vi "Initialise Tree.vi"(8 "error in (no error)":errorcluster, 11 "Resource Directory":path) -> (0 "error out":errorcluster, 3 "Teapot":T1)   [LabVIEW 2022 SP3, in "Application.lvlib" / "Scene.lvclass"]
uses:
  Scene.lvclass
  Libraries/3D/Object.ctl
  Libraries/3D/Triangle 3D.ctl
  Libraries/3D/Vector 3D.ctl
  Libraries/3D/Transform.ctl
  Libraries/3D/3D.lvlib
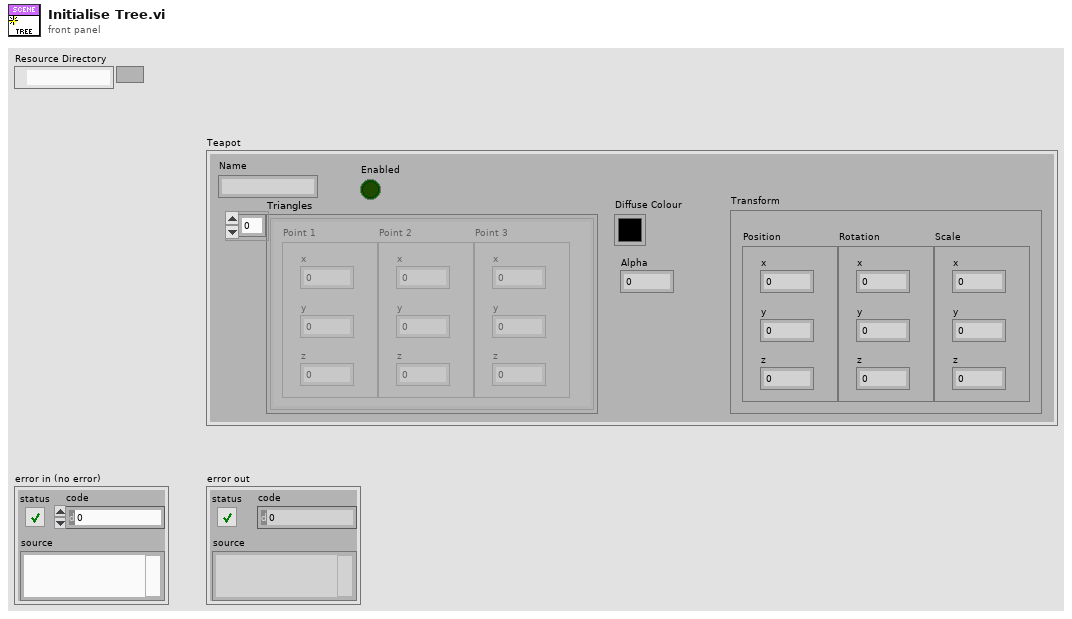
[diagram p1: front panel]
types:
  T1 = typedef "3D.lvlib/Object.ctl" = cluster{"Triangles":T2[], "Diffuse Colour":u32, "Transform":T4, "Name":string, "Enabled":bool, "Alpha":dbl}
  T2 = typedef "3D.lvlib/Triangle 3D.ctl" = cluster{"Point 1":T3, "Point 2":T3, "Point 3":T3}
  T3 = typedef "3D.lvlib/Vector 3D.ctl" = cluster{"x":sgl, "y":sgl, "z":sgl}
  T4 = typedef "3D.lvlib/Transform.ctl" = cluster{"Position":T3, "Rotation":T3, "Scale":T3}
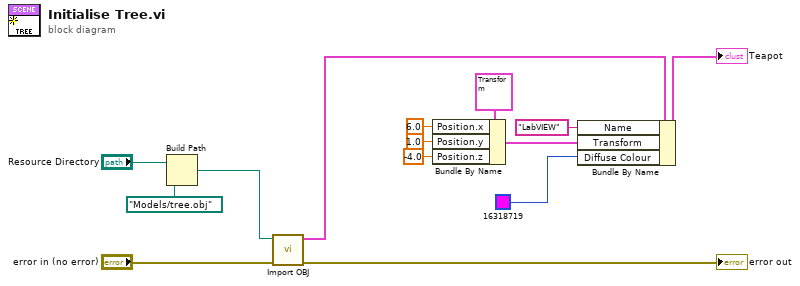
[diagram p0: block diagram]
diagram:
  n1 = Build Path(base path="Resource Directory", name or relative path=path "Models/tree.obj") -> (appended path=w3:path)
  n2 = call "Import OBJ.vi"("error in (no error)"="error in (no error)", "Object"=w3) -> ("error out"=→"error out":errorcluster, "Object"=w5:T1)  [unwired: 8 in]
  n3 = Bundle By Name(cluster=T4 {"Position"={"x"=2.0, "y"=1.0, "z"=-5.0}, "Rotation"={"x"=0.0, "y"=0.0, "z"=0.0}, "Scale"={"x"=0.0, "y"=0.0, "z"=0.0}} ("Transform"), "Position.x"=sgl 6.0, "Position.y"=sgl 1.0, "Position.z"=sgl -4.0) -> (w8:T4)
  n4 = Bundle By Name(cluster=w5, "Name"="LabVIEW", "Transform"=w8, "Diffuse Colour"=u32 16318719) -> (→"Teapot":T1)
